vi "eventos2.vi"() -> ()   [LabVIEW 2011]
panel:
  out "Led2":bool
  out "Encendido":dbl
  in  "salir":bool
  out "Led1":bool
  in  "Encender":bool
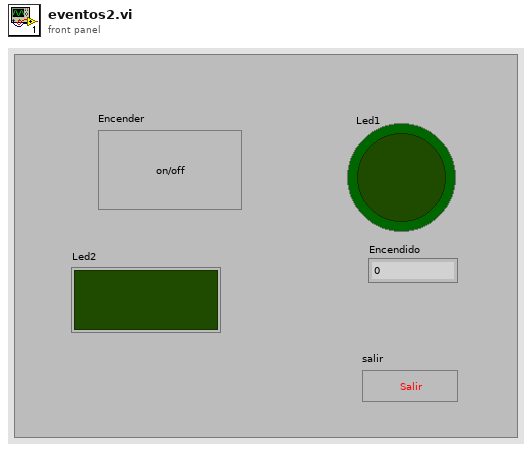
[diagram p1: front panel]
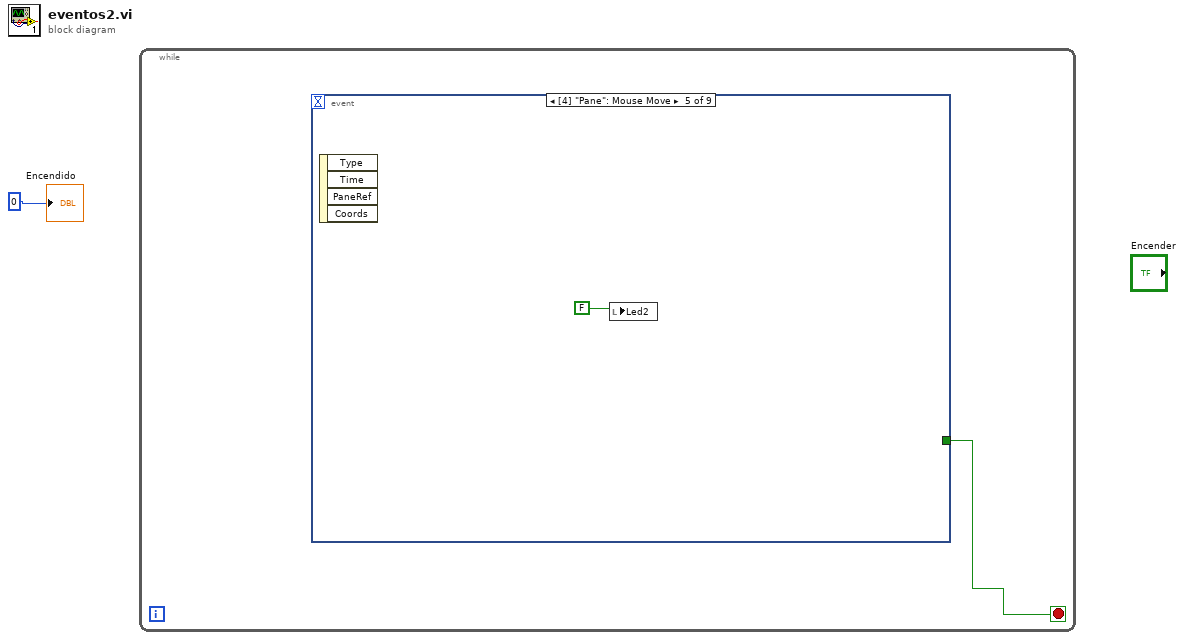
[diagram p0: block diagram]
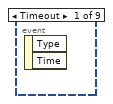
[diagram p2: hidden frame]
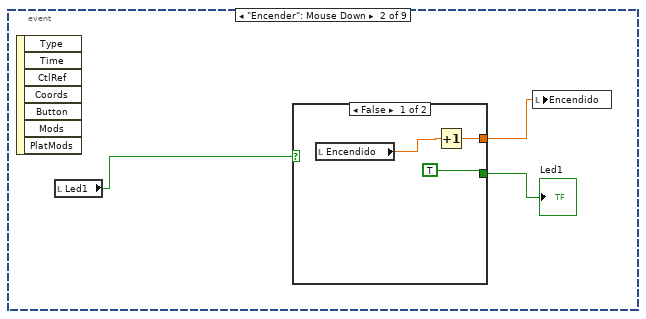
[diagram p3: hidden frame]
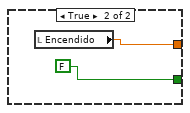
[diagram p4: hidden frame]
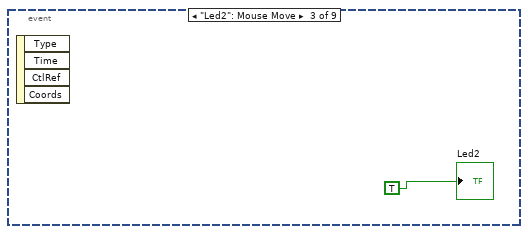
[diagram p5: hidden frame]
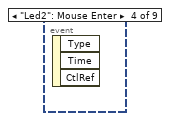
[diagram p6: hidden frame]
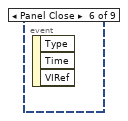
[diagram p7: hidden frame]
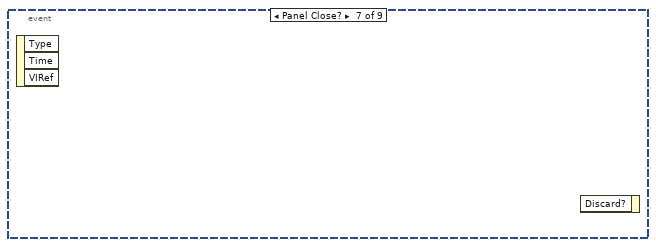
[diagram p8: hidden frame]
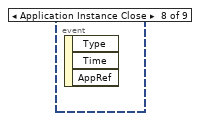
[diagram p9: hidden frame]
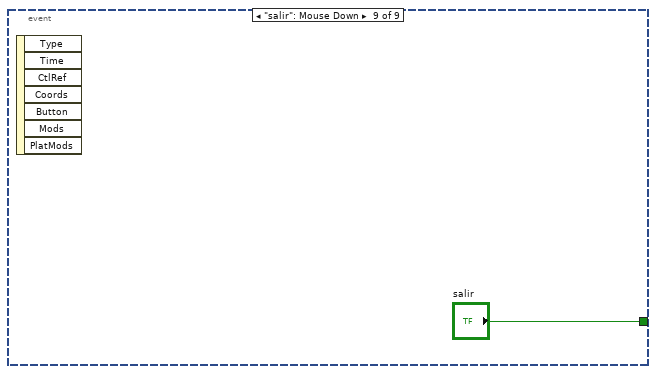
[diagram p10: hidden frame]
diagram:
  n1 = while {
    stop <- w2 stop-if-true
    n2 = event shown="[4] \"Pane\": Mouse Move" {
      selector: _ -> [_ _ _ _ _ _ _ _ _]
      dyn-events: _ -> [_ _ _ _ _ _ _ _ _]
      timeout: _ -> [_ _ _ _ _ _ _ _ _]
      tunnel: [_ _ _ _ _ _ _ _ "salir"] -> w2
      event Timeout {
        n3 = event-data() -> ()  [unwired: 1 in, 2 out]
      }
      event "Encender": Mouse Down {
        n4 = event-data() -> ()  [unwired: 1 in, 7 out]
        n5 = local read "Led1"() -> (w5:bool)
        n6 = case shown="False" w5 {
          tunnel: [TRUE FALSE] -> w4
          tunnel: [w6 w9] -> w3
          frame False {
            n7 = local read "Encendido"() -> (w7:dbl)
            n8 = Increment(x=w7) -> (x+1=w6:dbl)
          }
          frame True {
            n9 = local read "Encendido"() -> (w9:dbl)
          }
        }
        "Led1" <- w4
        n10 = local write "Encendido"(w3) -> ()
      }
      event "Led2": Mouse Move {
        n11 = event-data() -> ()  [unwired: 1 in, 4 out]
        "Led2" <- TRUE
      }
      event "Led2": Mouse Enter {
        n12 = event-data() -> ()  [unwired: 1 in, 3 out]
      }
      event Mouse Move {
        n13 = event-data() -> ()  [unwired: 1 in, 4 out]
        n14 = local write "Led2"(FALSE) -> ()
      }
      event Panel Close {
        n15 = event-data() -> ()  [unwired: 1 in, 3 out]
      }
      event Panel Close? {
        n16 = event-data() -> ()  [unwired: 1 in, 3 out]
        n17 = event-data() -> ()  [unwired: 2 in, 1 out]
      }
      event Application Instance Close {
        n18 = event-data() -> ()  [unwired: 1 in, 3 out]
      }
      event "salir": Mouse Down {
        n19 = event-data() -> ()  [unwired: 1 in, 7 out]
      }
    }
  }
  "Encendido" <- 0
